vi "OutTrigP.vi"() -> ()   [LabVIEW 2014]
uses:
  ESLSCDLL.dll
panel:
  in  "Numerisch":u32
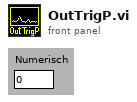
[diagram p1: front panel]
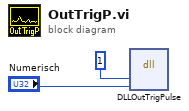
[diagram p0: block diagram]
diagram:
  n1 = dll-call lib="C:/Users/Gerhard/Documents/New64/lv/1cam/board.vis/ESLSCDLL.dll" fn="DLLOutTrigPulse"("drv"=u32 1, "PulseWidth"="Numerisch") -> ()  [unwired: 6 in, 2 out]
